vi "PC_SVG to DC-RMSM no trigger.vi"() -> ()   [LabVIEW 2021]
uses:
  Signal Voltage Generation/Typedefs/Signal Generation Settings.ctl
  Signal Voltage Generation/Typedefs/Generation Types.ctl
  Signal Voltage Generation/Typedefs/Single Tone Settings.ctl
  Signal Voltage Generation/Typedefs/Waveform Type.ctl
  Signal Voltage Generation/Typedefs/Tone Settings.ctl
  DC-RMS Voltage Measurement/Typedefs/DC and RMS Voltage Measurements.ctl
  Signal Voltage Generation/DAQ_Signal Voltage Generation.lvlib
  DC-RMS Voltage Measurement/DAQ_DC-RMS Voltage Measurement.lvlib
panel:
  out "Voltage Waveforms":waveform(dbl)[](graph)=[{"t0"=timestamp(3825153635.0917363 s since 1904-01-01), "dt"=9.999999999999999e-05, "Y"=array[1000 elements], "attributes"=variant("NI_ChannelName"=variant(string "Dev1/ai0"), "NI_UnitDescription"=variant(string "Volts"))}, {"t0"=timestamp(3825153635.0917473 s since 1904-01-01), "dt"=9.999999999999999e-05, "Y"=array[1000 elements], "attributes"=variant("NI_ChannelName"=variant(string "Dev1/ai1"), "NI_UnitDescription"=variant(string "Volts"))}, {"t0"=timestamp(3825153635.0917583 s since 1904-01-01), "dt"=9.999999999999999e-05, "Y"=array[1000 elements], "attributes"=variant("NI_ChannelName"=variant(string "Dev1/ai2"), "NI_UnitDescription"=variant(string "Volts"))}, {"t0"=timestamp(3825153635.091769 s since 1904-01-01), "dt"=9.999999999999999e-05, "Y"=array[1000 elements], "attributes"=variant("NI_ChannelName"=variant(string "Dev1/ai3"), "NI_UnitDescription"=variant(string "Volts"))}, {"t0"=timestamp(3825153635.09178 s since 1904-01-01), "dt"=9.999999999999999e-05, "Y"=array[1000 elements], "attributes"=variant("NI_ChannelName"=variant(string "Dev1/ai4"), "NI_UnitDescription"=variant(string "Volts"))}]
  out "DC-RMS Voltage Measurements":T1={"Average DC Voltage (V)"=[0.4994641302503497, 0.4993729245431572, 0.49941063149686055, 0.24917473308005667, 0.24822271311629407], "RMS Voltage (V)"=[0.6119366525415012, 0.6118729868071107, 0.6118748506601979, 0.30539901947038545, 0.30426490464326916]} caption="DC Voltage Measurements" {"RMS Voltage (V)" format="%.2p"; "Average DC Voltage (V)" format="%.2p"}
  out "Generated Voltage Waveforms":waveform(dbl)[](graph)=[{"t0"=timestamp(0 s since 1904-01-01), "dt"=1e-05, "Y"=array[20000 elements]}, {"t0"=timestamp(0 s since 1904-01-01), "dt"=1e-05, "Y"=array[20000 elements]}, {"t0"=timestamp(0 s since 1904-01-01), "dt"=1e-05, "Y"=array[20000 elements]}, {"t0"=timestamp(0 s since 1904-01-01), "dt"=1e-05, "Y"=array[20000 elements]}]
  in  "Signal Generation Settings":T2={"Generation Type"=enum."Single Tone", "Generation Time (s)"=0.2, "Voltage Offset (v)"=0.5, "Single Tone Settings"={"Waveform Type"=enum."Sine Wave", "Frequency (Hz)"=100.0, "Amplitude (V)"=0.5, "Duty Cycle (%)"=50.0}, "Multi Tone Settings"=[]} {"Voltage Offset (v)" format="%.2p"; "Generation Time (s)" format="%.2p"; "Multi Tone Settings"."Amplitude (V)" format="%#.2p"; "Multi Tone Settings"."Frequency (Hz)" format="%#.2p"; "Single Tone Settings"."Duty Cycle (%)" format="%#.2p"; "Single Tone Settings"."Amplitude (V)" format="%#.2p"; "Single Tone Settings"."Frequency (Hz)" format="%#.2p"}
  out "error out":errorcluster
  # "Frequency (Hz)"
  # "Amplitude (V)"
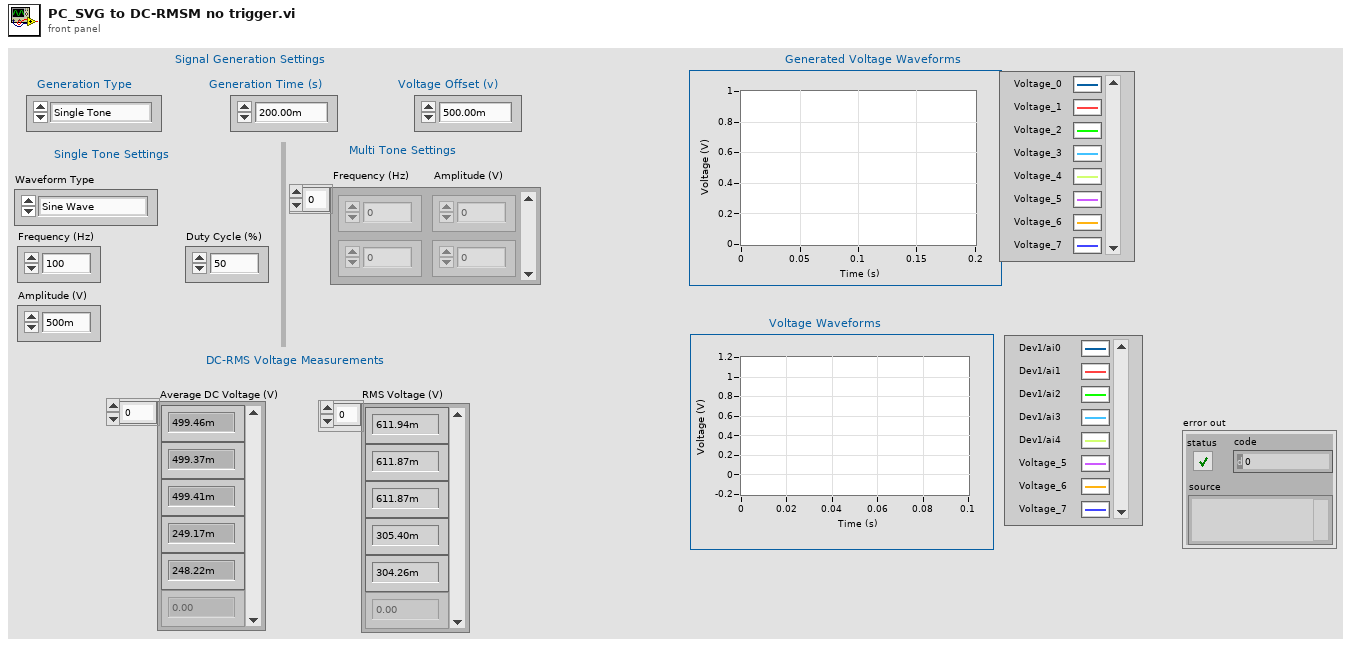
[diagram p1: front panel]
types:
  T1 = typedef "DAQ_DC-RMS Voltage Measurement.lvlib/DC and RMS Voltage Measurements.ctl" = cluster{"Average DC Voltage (V)":dbl[], "RMS Voltage (V)":dbl[]}
  T2 = typedef "DAQ_Signal Voltage Generation.lvlib/Signal Generation Settings.ctl" = cluster{"Generation Type":T3, "Generation Time (s)":dbl, "Voltage Offset (v)":dbl, "Single Tone Settings":T4, "Multi Tone Settings":T6[]}
  T3 = typedef "DAQ_Signal Voltage Generation.lvlib/Generation Types.ctl" = enum16{"Single Tone", "Multi Tone"}
  T4 = typedef "DAQ_Signal Voltage Generation.lvlib/Single Tone Settings.ctl" = cluster{"Waveform Type":T5, "Frequency (Hz)":dbl, "Amplitude (V)":dbl, "Duty Cycle (%)":dbl}
  T5 = typedef "DAQ_Signal Voltage Generation.lvlib/Waveform Type.ctl" = enum16{"Sine Wave", "Square Wave"}
  T6 = typedef "DAQ_Signal Voltage Generation.lvlib/Tone Settings.ctl" = cluster{"Frequency (Hz)":dbl, "Amplitude (V)":dbl}
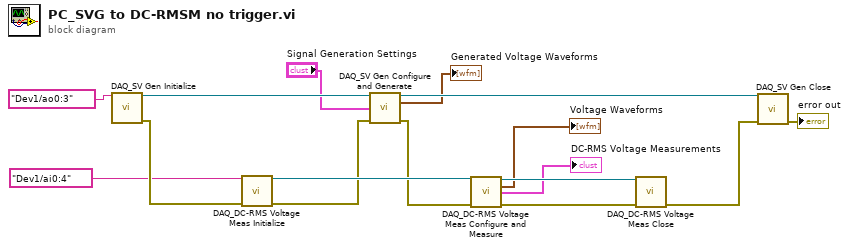
[diagram p0: block diagram]
diagram:
  n1 = call "DAQ_SV Gen Initialize.vi"("Physical Channels"=tag "Dev1/ao0:3") -> ("DAQmx Task Out"=w16:refnum<k21>, "error out"=w11:errorcluster)  [unwired: 13 in]
  n2 = call "DAQ_DC-RMS Voltage Meas Initialize.vi"("Physical Channels"=tag "Dev1/ai0:4", "error in"=w11) -> ("DAQmx Task Out"=w10:refnum<k21>, "error out"=w9:errorcluster)  [unwired: 12 in]
  n3 = call "DAQ_SV Gen Configure and Generate.vi"("DAQmx Task In"=w16, "Signal Generation Settings"="Signal Generation Settings", "error in"=w9) -> ("DAQmx Task Out"=w15:refnum<k21>, "Generated Voltage Waveforms"=→"Generated Voltage Waveforms":waveform(dbl)[], "error out"=w8:errorcluster)  [unwired: 10 in]
  n4 = call "DAQ_DC-RMS Voltage Meas Configure and Measure.vi"("DAQmx Task In"=w10, "error in"=w8) -> ("DAQmx Task Out"=w5:refnum<k21>, "Voltage Waveforms"=→"Voltage Waveforms":waveform(dbl)[], "DC and RMS Voltage Measurements"=→"DC-RMS Voltage Measurements":T1, "error out"=w7:errorcluster)  [unwired: 9 in, 1 out]
  n5 = call "DAQ_DC-RMS Voltage Meas Close.vi"("DAQmx Task In"=w5, "error in"=w7) -> ("error out"=w6:errorcluster)  [unwired: 13 in]
  n6 = call "DAQ_SV Gen Close.vi"("DAQmx Task In"=w15, "error in"=w6) -> ("error out"=→"error out":errorcluster)  [unwired: 13 in]
